vi "UDP dSpace Sender.vi"(6 "ENQUE DIRECTLY":refnum<queue>, 7 "milliseconds to wait":u32, 8 "error in (no error)":errorcluster, 9 "destination adress":string, 10 "destination port":u16, 11 "UDP Network Connection in":refnum<k16>) -> (0 "error out":errorcluster)   [LabVIEW 2016]
uses:
  Globale Variablen VI/Global Variables.vi
  Globale Variablen VI/RadSensoren.vi
  Globale Variablen VI/AutonomousMode.vi
panel:
  out "ss":dbl
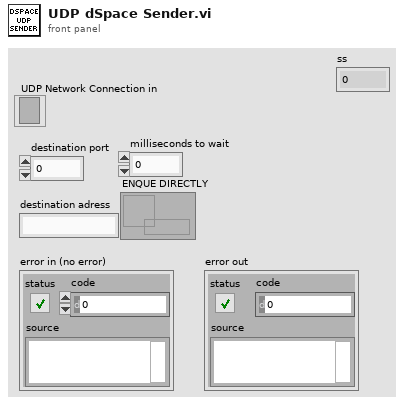
[diagram p1: front panel]
types:
  T1 = enum16{"big-endian, network order", "native, host order", "little-endian"}
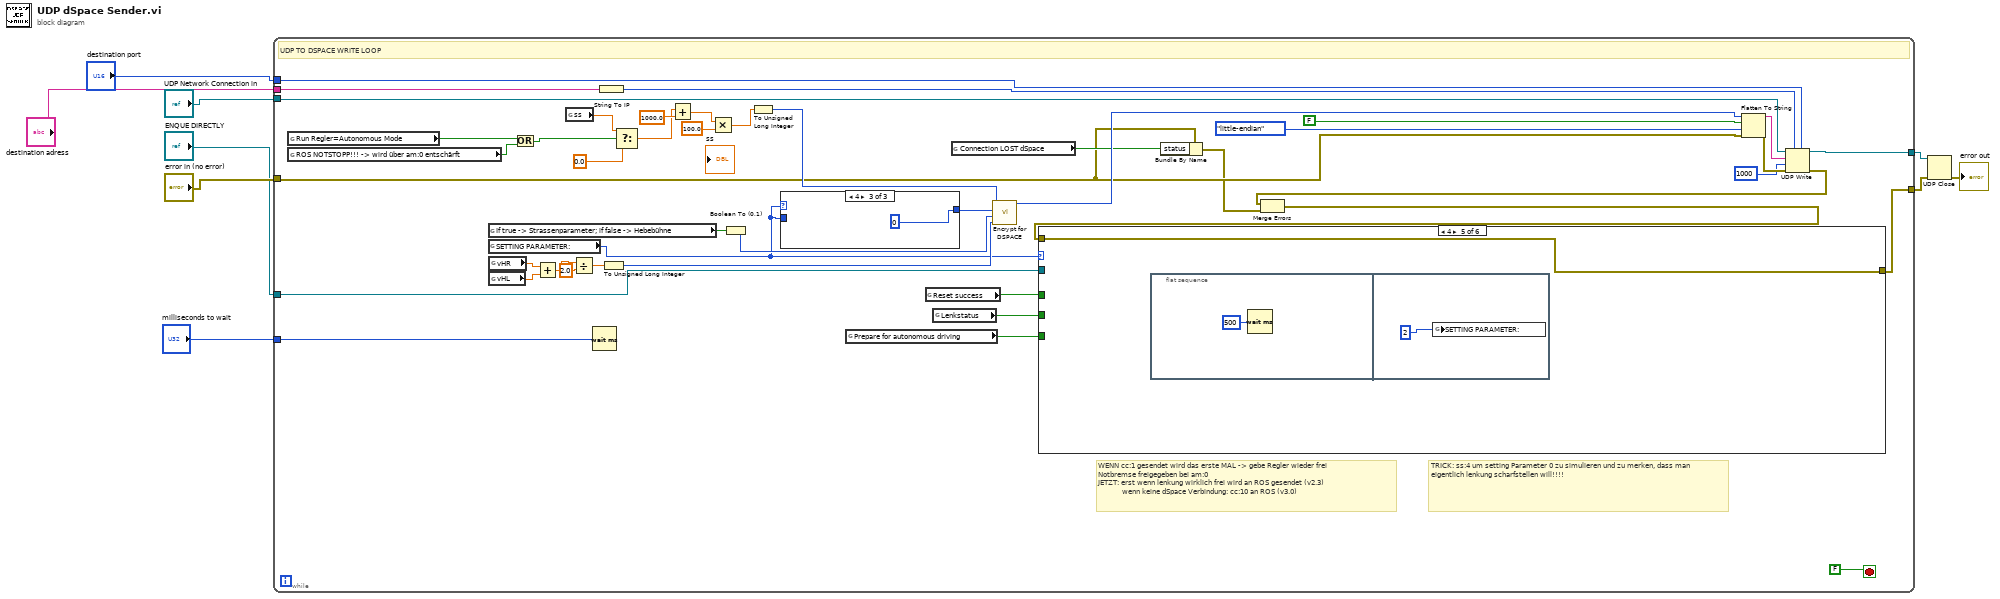
[diagram p0: block diagram]
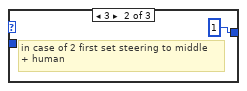
[diagram p3: hidden frame]
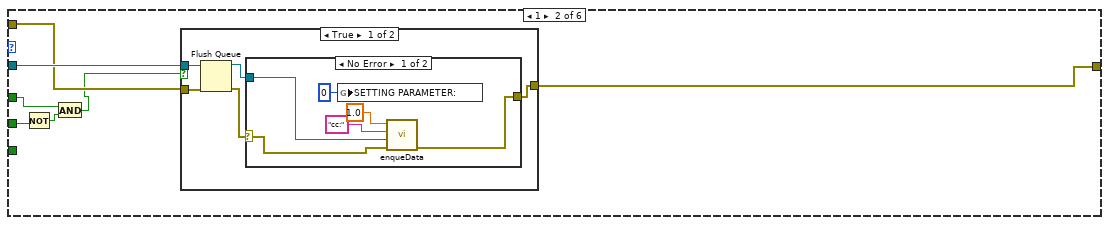
[diagram p5: hidden frame]
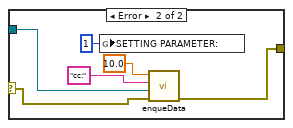
[diagram p6: hidden frame]
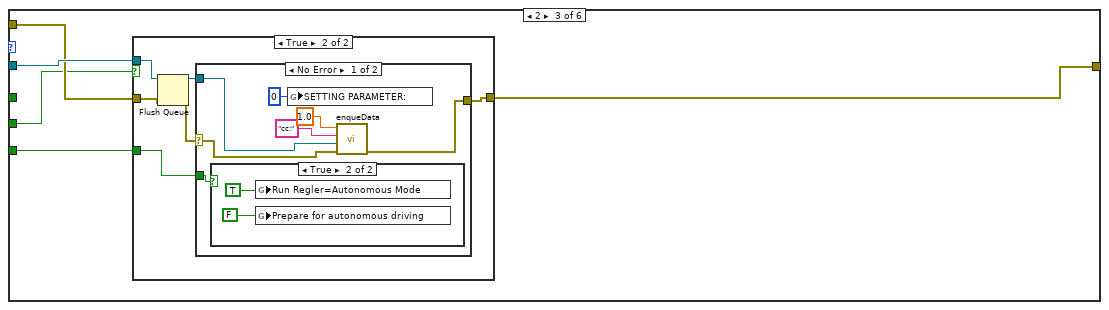
[diagram p8: hidden frame]
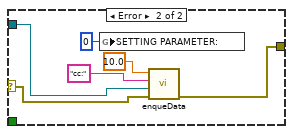
[diagram p11: hidden frame]
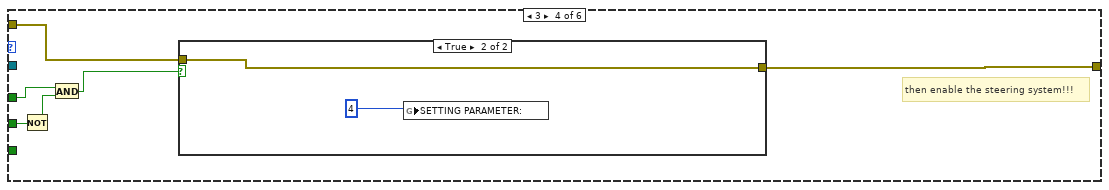
[diagram p12: hidden frame]
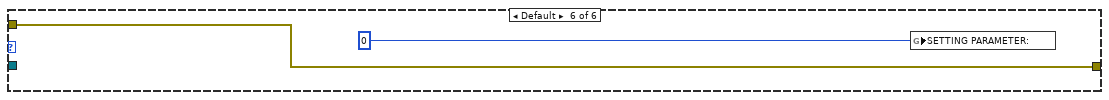
[diagram p14: hidden frame]
diagram:
  n1 = while {
    tunnel: [w36] -> w6
    tunnel: [w53] -> w7
    tunnel: "error in (no error)" -> [w25]
    tunnel: "UDP Network Connection in" -> [w52]
    tunnel: "destination port" -> [w51]
    tunnel: "destination adress" -> [w47]
    tunnel: "milliseconds to wait" -> [w44]
    tunnel: "ENQUE DIRECTLY" -> [w29]
    stop <- FALSE stop-if-true
    # "TRICK: ss:4 um setting Parameter 0 zu simulieren und zu merken, dass man eigentlich lenkung scharfstellen will!!!!"
    # "WENN cc:1 gesendet wird das erste MAL -> gebe Regler wieder frei\nNotbremse freigegeben bei am:0\nJETZT: erst wenn lenkung wirklich frei wird an ROS gesendet (v2.3)\n            wenn keine dSpace Verbindung: cc:10 an ROS (v3.0)"
    # "UDP TO DSPACE WRITE LOOP"
    n2 = global read "AutonomousMode.vi" "Run Regler=Autonomous Mode"() -> (w11:bool)
    n3 = global read "AutonomousMode.vi" "ROS NOTSTOPP!!! -> wird über am:0 entschärft"() -> (w12:bool)
    n4 = global read "AutonomousMode.vi" "If true -> Strassenparameter; if false -> Hebebühne"() -> (w37:bool)
    n5 = global read "Global Variables.vi" "SETTING PARAMETER:"() -> (w31:i32)
    n6 = global read "RadSensoren.vi" "vHR"() -> (w41:sgl)
    n7 = global read "RadSensoren.vi" "vHL"() -> (w42:sgl)
    n8 = Or(x=w11, y=w12) -> (x .or. y?=w10:bool)
    n9 = Add(x=w41, y=w42) -> (x+y=w40:sgl)
    n10 = global read "Global Variables.vi" "ss"() -> (w15:dbl)
    n11 = Divide(x=w40, y=sgl 2.0) -> (x/y=w38:sgl)
    n12 = Wait (ms)(milliseconds to wait=w44) -> ()  [unwired: 1 out]
    n13 = String To IP(1:w47) -> (0:w46:u32)
    n14 = To Unsigned Long Integer(number=w38) -> (unsigned 32bit integer=w33:u32)
    n15 = Select(t=w15, s=w10, f=0.0) -> (s? t:f=w14:dbl)
    n16 = Add(x=w14, y=1000.0) -> (x+y=w18:dbl)
    n17 = Multiply(x=w18, y=100.0) -> (x*y=w20:dbl)
    n18 = Boolean To (0,1)(Boolean=w37) -> (0, 1=w34:i16)
    n19 = To Unsigned Long Integer(number=w20) -> (unsigned 32bit integer=w35:u32)
    n20 = case shown="4" w31 {
      tunnel: w31 -> [w54 _ _]
      tunnel: [w54 1 0] -> w30
      frame Default {
      }
      frame 3 {
        # "in case of 2 first set steering to middle \n+ human"
      }
      frame 4 {
      }
    }
    n21 = global read "AutonomousMode.vi" "Prepare for autonomous driving"() -> (w16:bool)
    n22 = global read "Global Variables.vi" "Reset success"() -> (w27:bool)
    n23 = global read "Global Variables.vi" "Lenkstatus"() -> (w17:bool)
    n24 = global read "Global Variables.vi" "Connection LOST dSpace"() -> (w26:bool)
    n25 = call "Encrypt for DSPACE.vi"("ss"=w35, "SETTING PARAMETER:"=w30, "Hebe or Street"=w34, "velocity"=w33) -> ("Message for dSpace"=w32:u32)  [unwired: 6 in]
    n26 = Bundle By Name(cluster=w25, "status"=w26) -> (w24:errorcluster)
    n27 = Flatten To String(anything=w32, prepend array or string size? (T)=FALSE, byte order (0:big-endian, network order)=T1."little-endian", error in (no error)=w25) -> (data string=w50:string, error out=w45:errorcluster)  [unwired: 1 out]
    n28 = UDP Write(address=w46, port or service name=w51, connection ID=w52, data in=w50, 8:w45, 9:1000 ("timeout ms (25000)")) -> (error out=w23:errorcluster, 3:w53:refnum<k16>)
    n29 = Merge Errors(w23, w24) -> (w22:errorcluster)
    n30 = case shown="4" w31 {
      tunnel: w22 -> [w57 w62 w86 w115 w119 w122]
      tunnel: w29 -> [_ w64 w87 _ _ _]
      tunnel: [w57 w63 w85 w114 w119 w122] -> w36
      tunnel: w27 -> [_ w59 _ w111 _ _]
      tunnel: w17 -> [_ w61 w84 w113 _ _]
      tunnel: w16 -> [_ _ w83 _ _ _]
      frame 0 {
      }
      frame 1 {
        n31 = Not(x=w61) -> (.not. x?=w60:bool)
        n32 = And(x=w59, y=w60) -> (x .and. y?=w58:bool)
        n33 = case shown="True" w58 {
          tunnel: w64 -> [w69 _]
          tunnel: [w65 w82] -> w63
          tunnel: w62 -> [w68 w82]
          frame True {
            n34 = Flush Queue(queue=w69, error in (no error)=w68) -> (queue out=w66:refnum<queue>, error out=w67:errorcluster)  [unwired: 1 out]
            n35 = case shown="No Error" w67 {
              selector: w67 -> [w72 w78]
              tunnel: [w71 w77] -> w65
              tunnel: w66 -> [w70 w76]
              frame No Error {
                n36 = global write "Global Variables.vi" "SETTING PARAMETER:"(0 ("SETTING PARAMETER:")) -> ()
                n37 = call "enqueData.vi"("error in (no error)"=w72, "Queue Reference"=w70, "Descriptor"="cc:", "Value IN"=1.0) -> ("error out"=w71:errorcluster)  [unwired: 7 in]
              }
              frame Error {
                n38 = global write "Global Variables.vi" "SETTING PARAMETER:"(1 ("SETTING PARAMETER:")) -> ()
                n39 = call "enqueData.vi"("error in (no error)"=w78, "Queue Reference"=w76, "Descriptor"="cc:", "Value IN"=10.0) -> ("error out"=w77:errorcluster)  [unwired: 7 in]
              }
            }
          }
          frame False {
          }
        }
      }
      frame 2 {
        n40 = case shown="True" w84 {
          tunnel: w87 -> [_ w94]
          tunnel: w86 -> [w88 w93]
          tunnel: [w88 w90] -> w85
          tunnel: w83 -> [_ w89]
          frame False {
          }
          frame True {
            n41 = Flush Queue(queue=w94, error in (no error)=w93) -> (queue out=w91:refnum<queue>, error out=w92:errorcluster)  [unwired: 1 out]
            n42 = case shown="No Error" w92 {
              selector: w92 -> [w97 w106]
              tunnel: w91 -> [w98 w105]
              tunnel: [w96 w104] -> w90
              tunnel: w89 -> [w95 _]
              frame No Error {
                n43 = case shown="True" w95 {
                  frame False {
                  }
                  frame True {
                    n44 = global write "AutonomousMode.vi" "Run Regler=Autonomous Mode"(TRUE) -> ()
                    n45 = global write "AutonomousMode.vi" "Prepare for autonomous driving"(FALSE) -> ()
                  }
                }
                n46 = global write "Global Variables.vi" "SETTING PARAMETER:"(0 ("SETTING PARAMETER:")) -> ()
                n47 = call "enqueData.vi"("error in (no error)"=w97, "Queue Reference"=w98, "Descriptor"="cc:", "Value IN"=1.0) -> ("error out"=w96:errorcluster)  [unwired: 7 in]
              }
              frame Error {
                n48 = global write "Global Variables.vi" "SETTING PARAMETER:"(0 ("SETTING PARAMETER:")) -> ()
                n49 = call "enqueData.vi"("error in (no error)"=w106, "Queue Reference"=w105, "Descriptor"="cc:", "Value IN"=10.0) -> ("error out"=w104:errorcluster)  [unwired: 7 in]
              }
            }
          }
        }
      }
      frame 3 {
        # "then enable the steering system!!!"
        n50 = Not(x=w113) -> (.not. x?=w112:bool)
        n51 = And(x=w111, y=w112) -> (x .and. y?=w110:bool)
        n52 = case shown="True" w110 {
          tunnel: w115 -> [w116 w118]
          tunnel: [w116 w118] -> w114
          frame False {
          }
          frame True {
            n53 = global write "Global Variables.vi" "SETTING PARAMETER:"(4) -> ()
          }
        }
      }
      frame 4 {
        n54 = flat-sequence {
          frame #0 {
            n55 = Wait (ms)(milliseconds to wait=u32 500) -> ()  [unwired: 1 out]
          }
          frame #1 {
            n56 = global write "Global Variables.vi" "SETTING PARAMETER:"(2) -> ()
          }
        }
      }
      frame Default {
        n57 = global write "Global Variables.vi" "SETTING PARAMETER:"(0 ("SETTING PARAMETER:")) -> ()
      }
    }
  }
  n58 = UDP Close(connection ID=w7, 8:w6) -> (error out=→"error out":errorcluster)  [unwired: 1 out]
